vi "EnableEqualization.vi"(8 "error in (no error)":errorcluster, 10 "Enable/Disable":bool, 11 "reference in":refnum<class "niMmWave_Transceiver.lvclass">) -> (0 "error out":errorcluster, 3 "reference out":refnum<class "niMmWave_Transceiver.lvclass">)   [LabVIEW 2019, in "niMmWave_Transceiver.lvclass"]
doc: "Enables or disabled signal calibration"
uses:
  niMmWave_Transceiver.lvclass
  C:/Barkhausen mmWave radar/Development/LV/Barkhausen mmWave hardware control/Host/SubVIs/mmWave instrument_class/mmWave instrument.lvclass
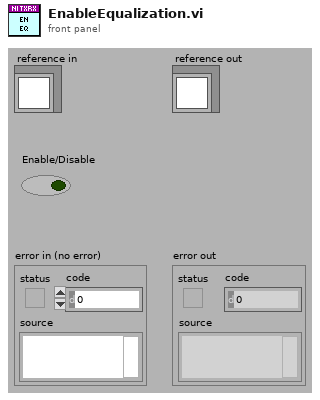
[diagram p1: front panel]
types:
  T1 = cluster{"I inline":dbl[], "I cross":dbl[], "Q cross":dbl[], "Q inline":dbl[]}
  T2 = typedef "niMmWave_Transceiver.lvclass/ObjectAttributesRef.ctl" = refnum<data-value>
  T3 = typedef "niMmWave_Transceiver.lvclass/ObjectAttributes.ctl" = cluster{"session":T4[], "HW.RX resources":T18, "RF config":T19, "RX trigger options":T20, "TX trigger options":T20, "RX samples":i32, "Downloaded Bursts":map{string, T23}, "TX Fs":dbl, "RX Fs":dbl, "burst sequence":string[]}
  T4 = typedef "Session.ctl" = cluster{"3620 session":refnum<queue>, "tx baseband session":T5, "rx baseband session":T13, "tx gain (dB)":dbl, "rx gain (dB)":dbl, "hardware configuration":T14, "gain ranging":T16[], "pxi trigger bus information":T17}
  T5 = typedef "Tx Baseband Session.ctl" = cluster{"3610 session":T6, "7902 reference":T12}
  T6 = typedef "ni3610_and_ni3630_Driver_Lib.lvlib/Main Settings.ctl" = cluster{"VISA resource name":refnum<visa-resource-name>, "Address Space":T7, "window_offset":u32, "register_addresses":T8, "required_MM_fpga_version":cluster{"signature":u32, "hardware":u32, "current revision":u32, "oldest revision":u32}, "CPLD Oldest Compat Version ":cluster{"hardware":u32, "CPLD firmware":u32}, "MM_FPGA_image_location":string, "is_init":bool, "card_type":T9, "DacLmkConfigFileName":string, "AdcLmkConfigFileName":string, "AdcConfigFileName":string, "DacConfigFileName_RevA":string, "DacConfigFileName_RevB":string, "Mulde hardware revision":u8, "bypass DAC PLL\n":bool, "IQ Card Revision":T10, "board capability":T11}
  T7 = typedef "VISA Register Access Address Space.ctl" = u16
  T8 = typedef "ni3610_and_ni3630_Driver_Lib.lvlib/Register Adresses.ctl" = cluster{"MM based Registers":cluster{"Revision":u32, "OldestCompatRev":u32, "signature":u32, "scratch":u32, "LedControl":u32, "BoardHwRev":u32, "BoardControl":u32, "ThermalStatus":u32, "BasebandStatus":u32, "BasebandControl":u32, "BasebandAuxSetup":u32, "BasebandAuxStatus":u32, "LmkSyncOutSetup":u32, " AdcSyncOutSetup":u32, " InjSyncOutSetup":u32, " PxiTrig0OutSetup":u32, " PxiTrig1OutSetup":u32, " PxiTrig2OutSetup":u32, " PxiTrig3OutSetup":u32, " PxiTrig4OutSetup":u32, " PxiTrig5OutSetup":u32, " PxiTrig6OutSetup":u32, " PxiTrig7OutSetup":u32}, "CPLD based Registers":cluster{"SlaveSignature":u32, "SlaveRevision":u32, "SlaveOldestCompatRev":u32, "SlaveScratch":u32, "SlaveSetup":u32, "SlaveStatus":u32, "IDacReg_offset":u32, "LMKRegGrp0_offset":u32, "QDacReg_offset":u32, "BrdTempSensorVal":u32, "TempSensorPowerDown":u32, "GPIOReg_offset":u32, "IAdcReg_offset":u32, "QAdcReg_offset":u32, "LMKRegGrp1_offset":u32, "QadcTempSensorVal":u32, "IadcTempSensorVal":u32, "RevisionReg":u32, "VcxoReg":u32, "CpldStatusReg":u32, "PowerReg":u32, "VBiasEnReg":u32, "ExtRefOeReg":u32, "QdacCtrlReg":u32, "QdacStatusReg":u32, "IdacCtrlReg":u32, "IdacStatusReg":u32, "QdacJtagIn":u32, "QdacJtagOut":u32, "IdacJtagIn":u32, "IdacJtagOut":u32, "IqDcSetupReg":u32, "QadcStatusReg":u32, "IadcStatusReg":u32, "BrdSetupReg":u32, "IqDcRevisionReg":u32, "PllStatusReg":u32, "EndpointScratchReg":u32, "AdcSyncCfgReg":u32, "IqCardOpampReg":u32}, "CPLD Register Offset":u32, "MM  Register Offset":u32, " PxiTrig0OutSetup":u32}
  T9 = typedef "ni3610_and_ni3630_Driver_Lib.lvlib/Base Card Type.ctl" = enum16{"unspecified", "ADC", "DAC"}
  T10 = typedef "ni3610_and_ni3630_Driver_Lib.lvlib/IQ Card Revision.ctl" = enum16{"RevA", "RevB", "RevC", "RevD"}
  T11 = typedef "ni3610_and_ni3630_Driver_Lib.lvlib/Board Capability.ctl" = cluster{"baseband sync":enum16{"no baseband sync", "baseband sync"}}
  T12 = typedef "Blank FPGA Reference.ctl" = refnum<k20>
  T13 = typedef "Rx Baseband Session.ctl" = cluster{"3630 session":T6, "7902 reference":T12}
  T14 = typedef "Hardware Configuration.ctl" = cluster{"direction":T15, "baseband only":bool}
  T15 = typedef "Direction.ctl" = enum16{"Transceiver", "Receiver", "Transmitter"}
  T16 = typedef "Gain Ranging.ctl" = cluster{"gain ranging active scope":string, "gain ranging stream session":refnum<k20>}
  T17 = typedef "PXI Trigger Bus Info.ctl" = cluster{"chassis resource name":refnum<visa-resource-name>, "7902R (TX)":i16, "3610 (TX)":i16, "3620 (IF)":i16, "3630 (RX)":i16, "7902R (RX)":i16}
  T18 = typedef "mmWave HW Control.lvlib/HW TXRX resources cluster.ctl" = cluster{"TX_DAC":refnum<visa-resource-name>, "TX_FPGA":tag, "IF":tag, "RX_ADC":refnum<visa-resource-name>, "RX_FPGA":tag}
  T19 = typedef "mmWave HW Control.lvlib/HW TXRX RF config cluster.ctl" = cluster{"TX.Frequency":dbl, "TX.Gain":dbl, "TX.mmWave adapter":string, "RX.Frequency":dbl, "RX.Gain":dbl, "RX.mmWave adapter":string}
  T20 = typedef "TX trigger config.ctl" = cluster{"delay":dbl, "trig source":T21, "PXI src":i32, "export":T22, "PXI dest":i32}
  T21 = typedef "FPGA Utility.lvlib/FPGA driver trigger source.ctl" = enum16{"Use Tclk", "PXI_Trig", "Aurora RX trig"}
  T22 = typedef "FPGA Utility.lvlib/FPGA driver trigger destination.ctl" = enum16{"None", "Source trig", "Synced trig", "Delayed sync"}
  T23 = typedef "niMmWave_Transceiver.lvclass/BurstInfo.ctl" = cluster{"starting addr":u32, "end addr":u32}
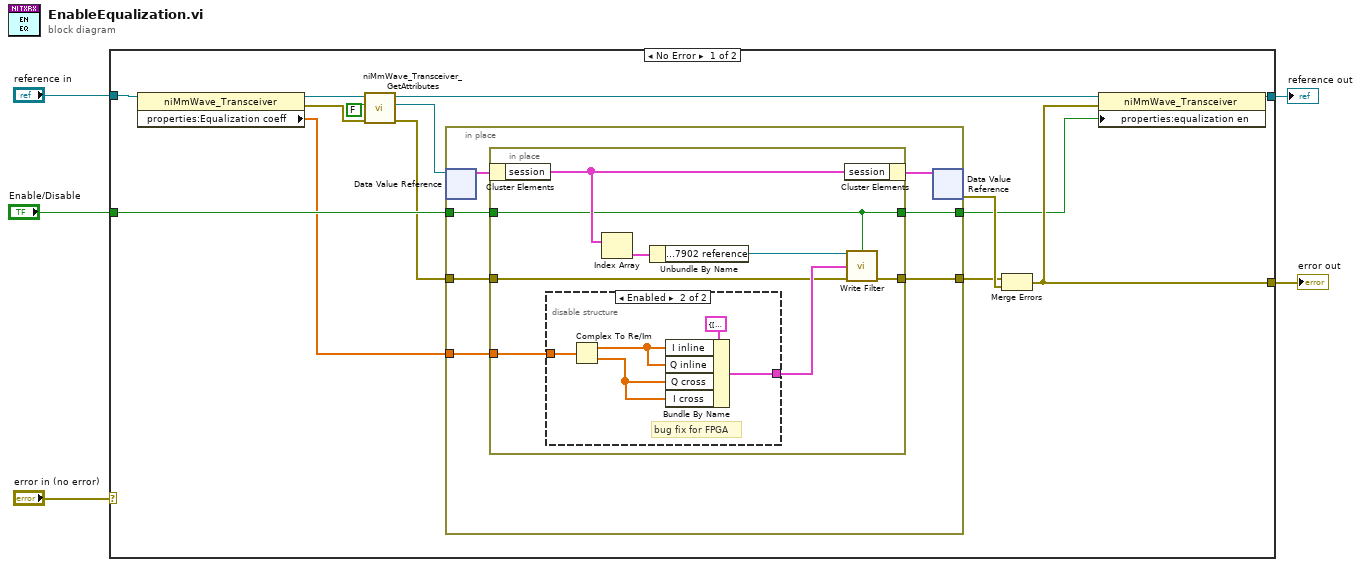
[diagram p0: block diagram]
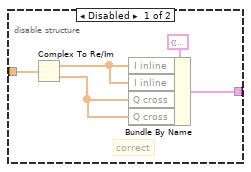
[diagram p2: hidden frame]
diagram:
  n1 = case shown="No Error" "error in (no error)" {
    selector: "error in (no error)" -> [_ w46]
    tunnel: [w7 w46] -> w4
    tunnel: [w8 w45] -> w2
    tunnel: "reference in" -> [w18 w45]
    tunnel: "Enable/Disable" -> [w14 _]
    frame No Error {
      n2 = property class="niMmWave_Transceiver"(reference=w18) -> (reference out=w13:refnum<class "niMmWave_Transceiver.lvclass">, error out=w11:errorcluster, "properties:Equalization coeff"=w12:cdb[])  [unwired: 1 in]
      n3 = call "niMmWave_Transceiver_GetAttributes.vi"("error in (no error)"=w11, "return data? (T)"=FALSE, "reference in"=w13) -> ("error out"=w10:errorcluster, "attributes ref"=w15:T2, "reference out"=w16:refnum<class "niMmWave_Transceiver.lvclass">)  [unwired: 5 in, 1 out]
      n4 = in-place {
        in-place-border: w14 -> [w24]
        in-place-border: w12 -> [w23]
        in-place-border: w10 -> [w22]
        in-place-border: [w21] -> w9
        in-place-border: [w20] -> w6
        n5 = in-place-dvr #1(w15) -> (w25:T3)  [unwired: 1 out]
        n6 = in-place {
          in-place-border: w24 -> [w27]
          in-place-border: w23 -> [w31]
          in-place-border: w22 -> [w29]
          in-place-border: [w28] -> w21
          in-place-border: [w27] -> w20
          n7 = in-place-cluster #2(w25) -> ("session"=w34:T4[])
          n8 = disable-structure shown="Enabled" {
            disable-tunnel: w31 -> [w39 w44]
            disable-tunnel: [w35 w40] -> w30
            frame Disabled {
              # "correct"
              n9 = Complex To Re/Im(x + iy=w39) -> (x=w37:dbl[], y=w36:dbl[])
              n10 = Bundle By Name(cluster=T1 {"I inline"=[], "I cross"=[], "Q cross"=[], "Q inline"=[]} ("coefficients"), "I inline"=w37, "I inline"=w37, "Q cross"=w36, "Q cross"=w36) -> (w35:T1)
            }
            frame Enabled {
              # "bug fix for FPGA"
              n11 = Complex To Re/Im(x + iy=w44) -> (x=w42:dbl[], y=w41:dbl[])
              n12 = Bundle By Name(cluster=T1 {"I inline"=[], "I cross"=[], "Q cross"=[], "Q inline"=[]} ("coefficients"), "I inline"=w42, "Q inline"=w42, "Q cross"=w41, "I cross"=w41) -> (w40:T1)
            }
          }
          n13 = Index Array(array=w34) -> (element=w33:T4)  [unwired: 1 in]
          n14 = Unbundle By Name(w33) -> ("rx baseband session.7902 reference"=w32:T12)
          n15 = in-place-cluster #2("session"=w34) -> (w26:T3)
          n16 = call "Write Filter.vi"("fpga reference in"=w32, "enable filter"=w27, "coefficients"=w30, "error in"=w29) -> ("error out"=w28:errorcluster)  [unwired: 10 in, 1 out]
        }
        n17 = in-place-dvr #1(w26) -> (w19:errorcluster)  [unwired: 1 out]
      }
      n18 = Merge Errors(w9, w19) -> (w7:errorcluster)
      n19 = property class="niMmWave_Transceiver"(reference=w16, error in=w7, "properties:equalization en"=w6) -> (reference out=w8:refnum<class "niMmWave_Transceiver.lvclass">)  [unwired: 1 out]
    }
    frame Error {
    }
  }
  "error out" <- w4
  "reference out" <- w2
